vi "Read Value.vi"(8 "error in (no error)":errorcluster, 11 "Bioreactor in":refnum<class "Bioreactor.lvclass">) -> (0 "error out":errorcluster, 3 "Bioreactor out":refnum<class "Bioreactor.lvclass">)   [LabVIEW 2012, in "Bioreactor Actor.lvlib" / "Bioreactor.lvclass"]
uses:
  Bioreactor.lvclass
  Bioreactor.lvclass/Bioreactor.ctl
  Read Address.vi
  Read VISA resource name.vi
  Read DVR.vi
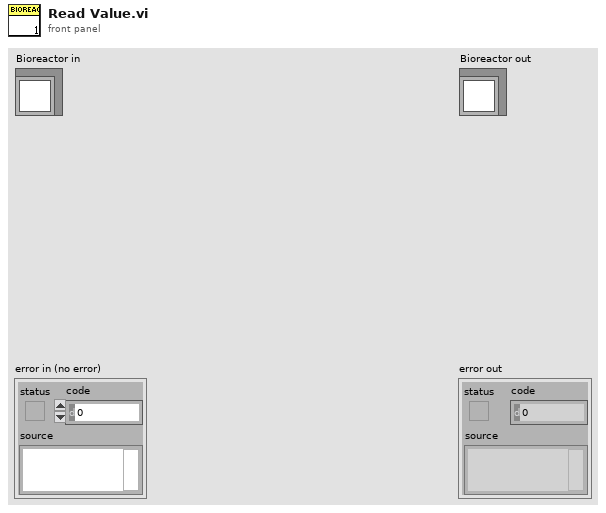
[diagram p1: front panel]
types:
  T1 = cluster{"Name":string, "Value":dbl, "Setpoint":dbl, "Output":dbl}[]
  T2 = cluster{"Name":string, "Value":dbl, "Setpoint":dbl, "Output":dbl}
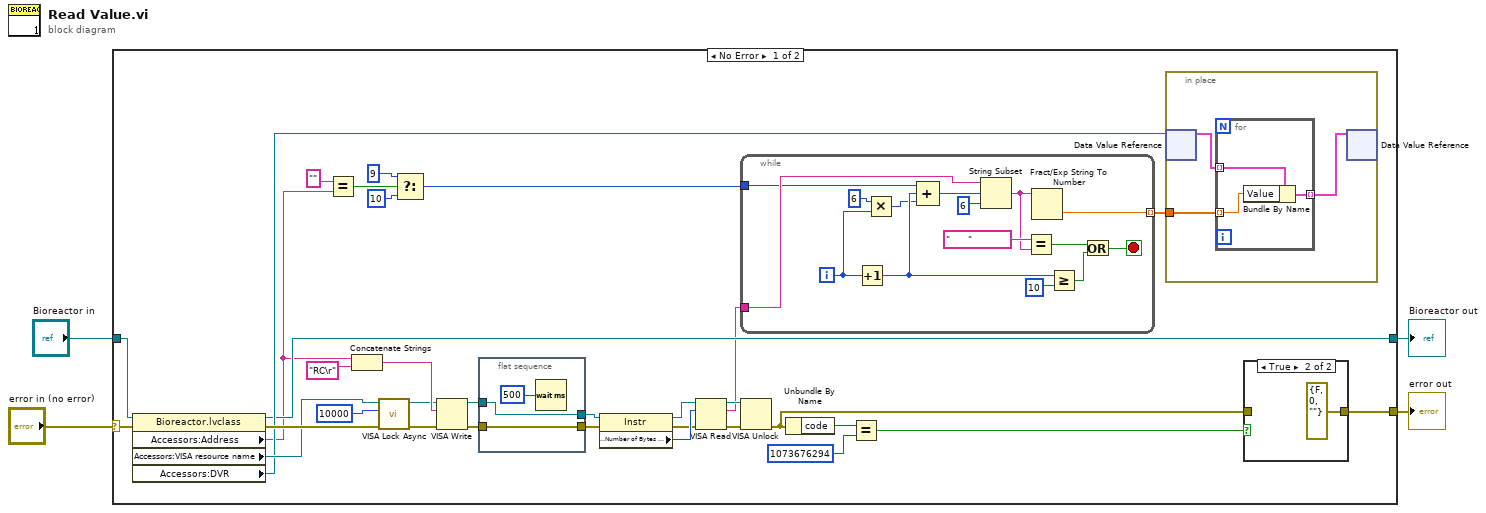
[diagram p0: block diagram]
diagram:
  n1 = case shown="No Error" "error in (no error)" {
    selector: "error in (no error)" -> [w25 w65]
    tunnel: [w14 w65] -> w3
    tunnel: [w13 w64] -> w1
    tunnel: "Bioreactor in" -> [w24 w64]
    frame No Error {
      n2 = property class="Bioreactor.lvclass"(reference=w24, error in=w25) -> (reference out=w13:refnum<class "Bioreactor.lvclass">, error out=w23:errorcluster, "Accessors:Address"=w6:string, "Accessors:VISA resource name"=w16:refnum<visa-resource-name>, "Accessors:DVR"=w15:refnum<data-value>)
      n3 = Equal?(x="", y=w6) -> (x = y?=w10:bool)
      n4 = Concatenate Strings(w6, "RC\r") -> (w29:string)
      n5 = call <vilib>:"VISA Lock Async.vi"("error in (no error)"=w23, "timeout (0)"=u32 10000, "VISA resource name"=w16) -> ("error out"=w22:errorcluster, "VISA resource name out"=w21:refnum<visa-resource-name>)  [unwired: 6 in, 1 out]
      n6 = Select(t=9, s=w10, f=10) -> (s? t:f=w5:i32)
      n7 = VISA Write(VISA resource name=w21, write buffer=w29, error in (no error)=w22) -> (VISA resource name out=w34:refnum<visa-resource-name>, error out=w32:errorcluster)  [unwired: 1 out]
      n8 = flat-sequence {
        tunnel: [w63] -> w33
        tunnel: w34 -> [w63]
        tunnel: [w62] -> w31
        tunnel: w32 -> [w62]
        frame #0 {
          n9 = Wait (ms)(milliseconds to wait=500 ("y")) -> ()  [unwired: 1 out]
        }
      }
      n10 = property class="Instr"(reference=w33, error in=w31) -> (reference out=w35:refnum<visa-resource-name>, error out=w36:errorcluster, "Serial Settings:Number of Bytes at Serial Port"=w37:u32)
      n11 = VISA Read(VISA resource name=w35, byte count=w37, error in (no error)=w36) -> (VISA resource name out=w17:refnum<visa-resource-name>, read buffer=w12:string, error out=w19:errorcluster)  [unwired: 1 out]
      n12 = while {
        tunnel: w12 -> [w52]
        tunnel: w5 -> [w51]
        tunnel: [w38] -> w11 mode=indexing
        i -> [w42]
        stop <- w45 stop-if-true
        n13 = Increment(x=w42) -> (x+1=w48:i32)
        n14 = Multiply(x=6, y=w42) -> (x*y=w41:i32)
        n15 = Compound Arithmetic op=ADD(w51, w48, w41) -> (w50:i32)
        n16 = String Subset(string=w52, offset (0)=w50, length (rest)=6) -> (substring=w39:string)
        n17 = Equal?(x="      " ("y"), y=w39) -> (x = y?=w49:bool)
        n18 = Fract/Exp String To Number(string=w39) -> (number=w38:dbl)  [unwired: 3 in, 1 out]
        n19 = Greater Or Equal?(x=w48, y=10) -> (x >= y?=w46:bool)
        n20 = Or(x=w49, y=w46) -> (x .or. y?=w45:bool)
      }
      n21 = VISA Unlock(8:w19, 11:w17) -> (0:w18:errorcluster)  [unwired: 1 out]
      n22 = Unbundle By Name(w18) -> ("code"=w28:i32)
      n23 = Equal?(x=w28, y=1073676294) -> (x = y?=w26:bool)
      n24 = in-place {
        in-place-border: w11 -> [w54]
        n25 = in-place-dvr #1(w15) -> (w55:T1)  [unwired: 1 out]
        n26 = for {
          tunnel: w55 -> [w58] mode=indexing
          tunnel: w54 -> [w57] mode=indexing
          tunnel: [w56] -> w53 mode=indexing
          n27 = Bundle By Name(cluster=w58, "Value"=w57) -> (w56:T2)
        }
        n28 = in-place-dvr #1(w53) -> ()  [unwired: 2 out]
      }
      n29 = case shown="True" w26 {
        tunnel: w18 -> [w59 _]
        tunnel: [w59 errorcluster {"status"=FALSE, "code"=0, "source"=""} ("error constant")] -> w14
        frame False {
        }
        frame True {
        }
      }
    }
    frame Error {
    }
  }
  "error out" <- w3
  "Bioreactor out" <- w1
